vi "URL_to_Variable.vi"(11 "URL":string="\\\\HousesOfTheHoly\\Leiden MNK\\Leiden MNK Front Panel\\MNK MF P_low") -> (3 "Name":string)   [LabVIEW 2019, in "data.citadel.lvclass"]
uses:
  data.citadel.lvclass
panel:
  out "after substring":string
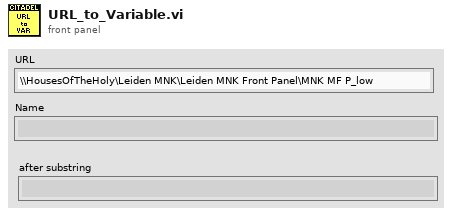
[diagram p1: front panel]
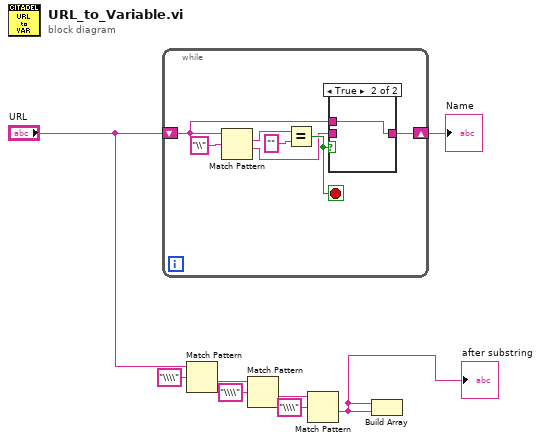
[diagram p0: block diagram]
diagram:
  n1 = while {
    shift-right: [w11] -> w8
    shift-left: "URL" -> [w9]
    stop <- w12 stop-if-true
    n2 = Match Pattern(string=w9, regular expression="\\") -> (match substring=w14:string, after substring=w10:string)  [unwired: 1 in, 2 out]
    n3 = Equal?(x=w14, y="" ("regular expression")) -> (x = y?=w12:bool)
    n4 = case shown="True" w12 {
      tunnel: [w16 w17] -> w11
      tunnel: w10 -> [w16 _]
      tunnel: w9 -> [_ w17]
      frame False {
      }
      frame True {
      }
    }
  }
  "Name" <- w8
  n5 = Match Pattern(string="URL", regular expression="\\\\") -> (after substring=w5:string)  [unwired: 1 in, 3 out]
  n6 = Match Pattern(string=w5, regular expression="\\\\") -> (after substring=w3:string)  [unwired: 1 in, 3 out]
  n7 = Match Pattern(string=w3, regular expression="\\\\") -> (after substring=w2:string)  [unwired: 1 in, 3 out]
  "after substring" <- w2
  n8 = Build Array(w2, w2) -> ()  [unwired: 1 out]
